vi "SA_INPUT_COUPLING.vi"(6 "AC/DC":enum16{"AC", "DC"}(ring), 8 "error in":errorcluster {"code" format="%.0x"}, 11 "Session In":refnum<visa-resource-name>="TCPIP0::K-N90X0A-00005.local::hislip0::INSTR") -> (0 "error out":errorcluster {"code" format="%.0x"}, 1 "Read":string, 3 "Session Out":refnum<visa-resource-name>)   [LabVIEW 2018]
doc: "This key does not appear in models that are always AC coupled. When the SCPI command to set\nDC coupling is sent to these models, it results in the error “Illegal parameter value; This model is\nalways AC coupled” In these models, the SCPI query INP:COUP? always returns AC.\nThis key does not appear in models that are always DC coupled.When the SCPI command to set\nAC coupling is sent to these models, it results in the error “Illegal parameter value; This\ninstrument is always DC coupled” In these models, the SCPI query INP:COUP? always returns DC."
panel:
  in  "Timeout":u32=3000
  in  "RO(T)":bool
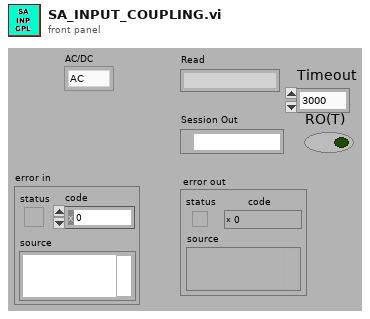
[diagram p1: front panel]
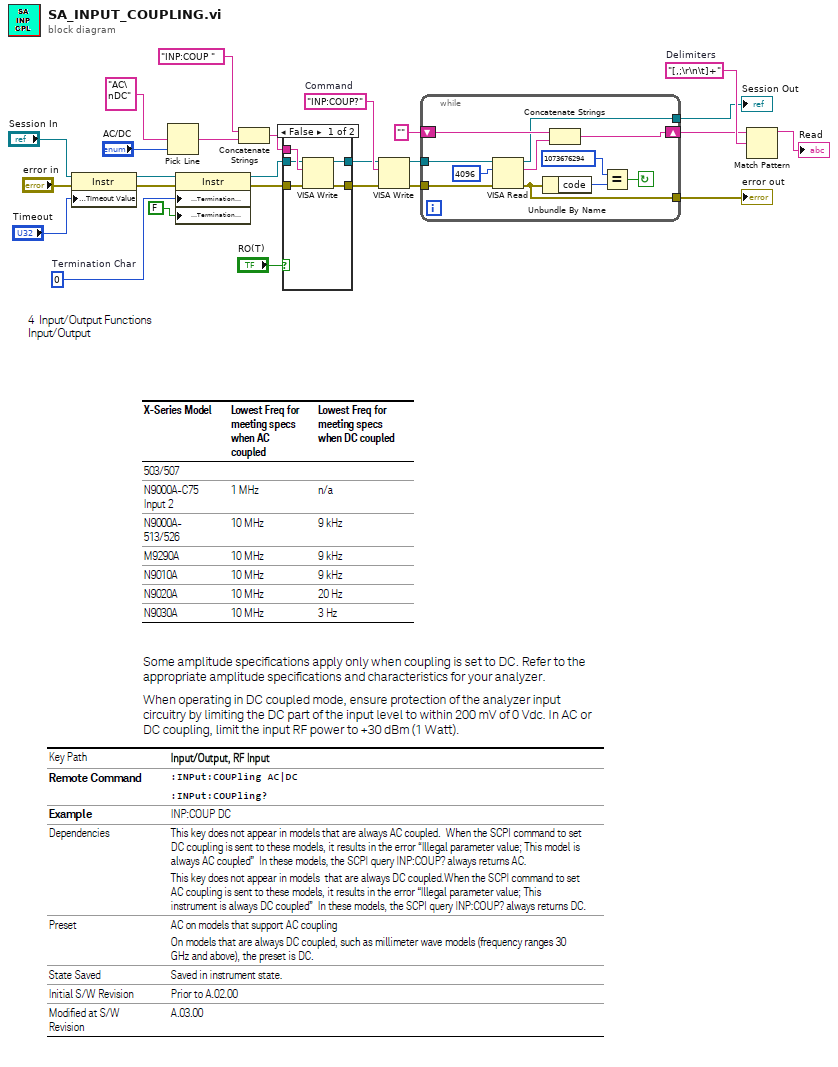
[diagram p0: block diagram]
diagram:
  w9 = "[,;\r\n\t]+"  # Delimiters
  w11 = "INP:COUP?"  # Command
  w21 = u8 0  # Termination Char
  n1 = property class="Instr"(reference="Session In", error in="error in", "General Settings:Timeout Value"="Timeout") -> (reference out=w20:refnum<visa-resource-name>, error out=w23:errorcluster)
  n2 = Pick Line(multi-line string="AC\nDC", line index="AC/DC") -> (output string=w1:string)  [unwired: 1 in]
  n3 = property class="Instr"(reference=w20, error in=w23, "Message Based Settings:Termination Character"=w21, "Message Based Settings:Termination Character Enable"=FALSE ("enable")) -> (reference out=w7:refnum<visa-resource-name>, error out=w22:errorcluster)
  n4 = Concatenate Strings("INP:COUP " ("staticText"), w1) -> (w16:string)
  n5 = case shown="False" "RO(T)" {
    tunnel: w22 -> [w31 w32]
    tunnel: [w30 w32] -> w17
    tunnel: w16 -> [w29 _]
    tunnel: w7 -> [w28 w33]
    tunnel: [w27 w33] -> w6
    frame False {
      n6 = VISA Write(VISA resource name=w28, write buffer=w29, error in (no error)=w31) -> (VISA resource name out=w27:refnum<visa-resource-name>, error out=w30:errorcluster)  [unwired: 1 out]
    }
    frame True {
    }
  }
  n7 = VISA Write(VISA resource name=w6, write buffer=w11, error in (no error)=w17) -> (VISA resource name out=w15:refnum<visa-resource-name>, error out=w14:errorcluster)  [unwired: 1 out]
  n8 = while {
    tunnel: w15 -> [w41]
    shift-right: [w35] -> w8
    shift-left: "" -> [w40]
    tunnel: w14 -> [w38]
    tunnel: [w37] -> w13
    tunnel: [w34] -> w5
    stop <- w36 continue-if-true
    n9 = VISA Read(VISA resource name=w41, byte count=u32 4096 ("byte count (0)"), error in (no error)=w38) -> (VISA resource name out=w34:refnum<visa-resource-name>, read buffer=w39:string, error out=w37:errorcluster)  [unwired: 1 out]
    n10 = Unbundle By Name(w37) -> ("code"=w43:i32)
    n11 = Concatenate Strings(w40, w39) -> (w35:string)
    n12 = Equal?(x=1073676294, y=w43) -> (x = y?=w36:bool)
  }
  "error out" <- w13
  "Session Out" <- w5
  n13 = Match Pattern(string=w8, regular expression=w9) -> (before substring=→"Read":string)  [unwired: 4 out]
